vi "Read datatype.vi"(8 "error in (no error)":errorcluster, 11 "JSON String in":refnum<class "JSON String.lvclass">) -> (0 "error out":errorcluster, 2 "datatype":T1, 3 "JSON String out":refnum<class "JSON String.lvclass">)   [LabVIEW 2015, in "LVJSON.lvlib" / "JSON String.lvclass"]
doc: "Returns the JSON Type of the given object. This may be used to determine if the value of a control of type JSON Null, JSON Literal or JSON Structured Type is an instance of a more specific type."
uses:
  JSON String.lvclass
  JSON Types.ctl
  LVJSON.lvlib
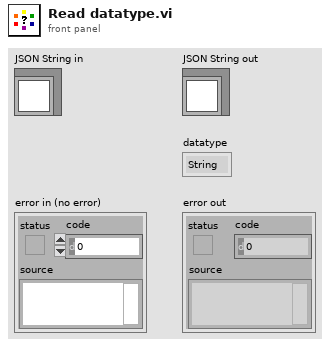
[diagram p1: front panel]
types:
  T1 = typedef "LVJSON.lvlib/JSON Types.ctl" = enum16{"String", "Numeric", "Boolean", "NULL", "Object", "Array"}
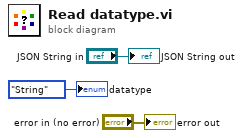
[diagram p0: block diagram]
diagram:
  "error out" <- "error in (no error)"
  "JSON String out" <- "JSON String in"
  "datatype" <- JSON_Types."String" ("datatype")
